vi "Filament Control.vi"(8 "error in (no error)":errorcluster, 9 "Filament":bool, 10 "Filament ID":i32, 11 "Pressure Monitor in":refnum<class "Pressure Monitor.lvclass">) -> (0 "error out":errorcluster, 3 "Pressure Monitor out":refnum<class "Pressure Monitor.lvclass">)   [LabVIEW 2024, in "Pressure Monitor.lvclass"]
uses:
  Pressure Monitor.lvclass
  Pressure Monitor.lvclass/Pressure Monitor.ctl
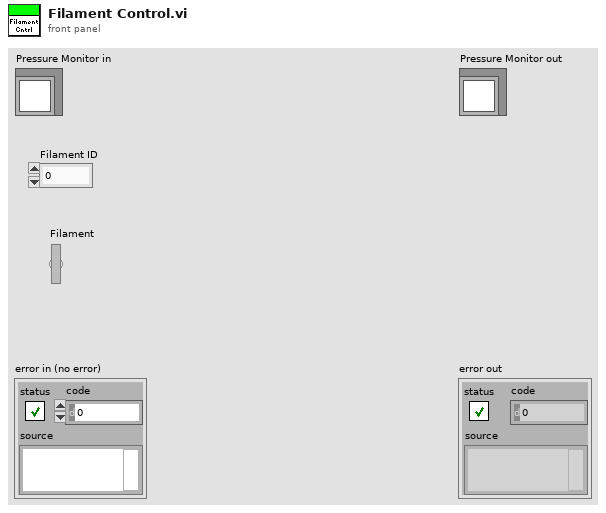
[diagram p1: front panel]
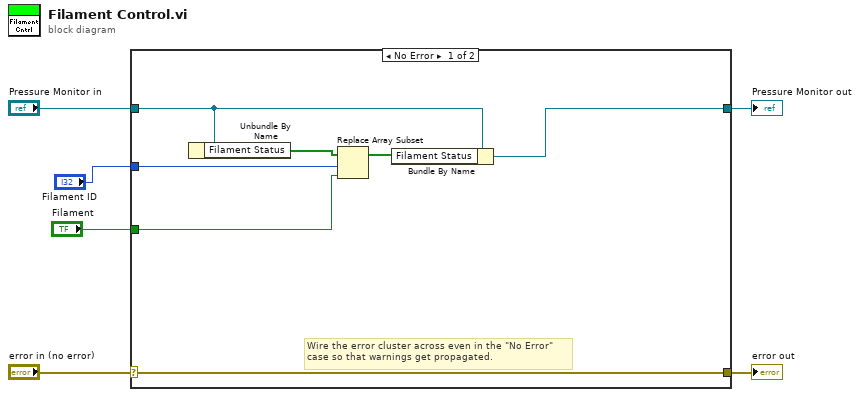
[diagram p0: block diagram]
diagram:
  n1 = case shown="No Error" "error in (no error)" {
    selector: "error in (no error)" -> [w13 w15]
    tunnel: [w13 w15] -> w5
    tunnel: [w8 w14] -> w3
    tunnel: "Pressure Monitor in" -> [w7 w14]
    tunnel: "Filament ID" -> [w11 _]
    tunnel: "Filament" -> [w10 _]
    frame No Error {
      # "Wire the error cluster across even in the \"No Error\"\ncase so that warnings get propagated."
      n2 = Unbundle By Name(w7) -> ("Filament Status"=w12:bool[])
      n3 = Replace Array Subset(array=w12, new element=w10, index=w11) -> (w9:bool[])
      n4 = Bundle By Name(cluster=w7, "Filament Status"=w9) -> (w8:refnum<class "Pressure Monitor.lvclass">)
    }
    frame Error {
    }
  }
  "error out" <- w5
  "Pressure Monitor out" <- w3
